vi "main.vi"() -> ()   [LabVIEW 2015]
uses:
  <vilib>/addons/InsightCM/MessageBus/MessageService/IcmMessageService.lvclass
  System/System.lvlib
  ConfigHelper/ConfigHelper.lvlib
  FileHandler/FileHandler.lvlib
  MainController/MainController.lvlib
  <vilib>/addons/Qbus/Qbus.lvclass
  CopyUtility/CopyUtility.lvlib
panel:
  in  "Control":bool
  out "System Status":string
  out "path":path
  out "error out":errorcluster
  out "Received Messages":i32(listbox)
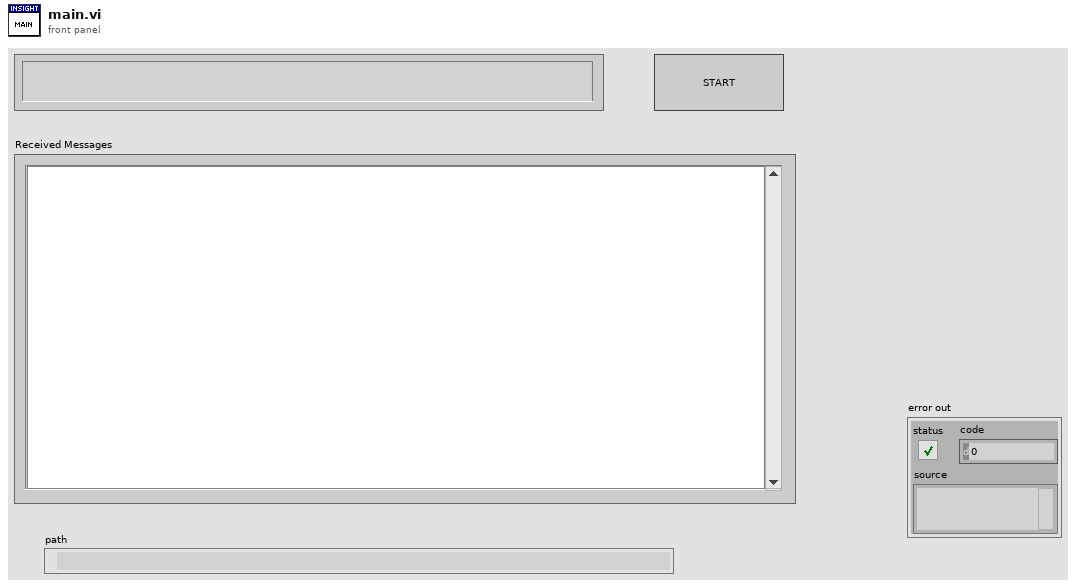
[diagram p1: front panel]
types:
  T1 = typedef "Message.ctl" = cluster{"Header":T2, "Body":u8[]}
  T2 = typedef "MessageHeader.ctl" = cluster{"MessageName":string, "Timestamp":i64, "CorrelationId":string, "ContentType":string, "RoutingKey":string, "Properties":T3[]}
  T3 = typedef "KeyValuePair.ctl" = cluster{"Key":string, "Value":string}
  T4 = typedef "StorageFileAvailableBroadcastBody.ctl" = cluster{"DeviceName":string, "Filepath":string}
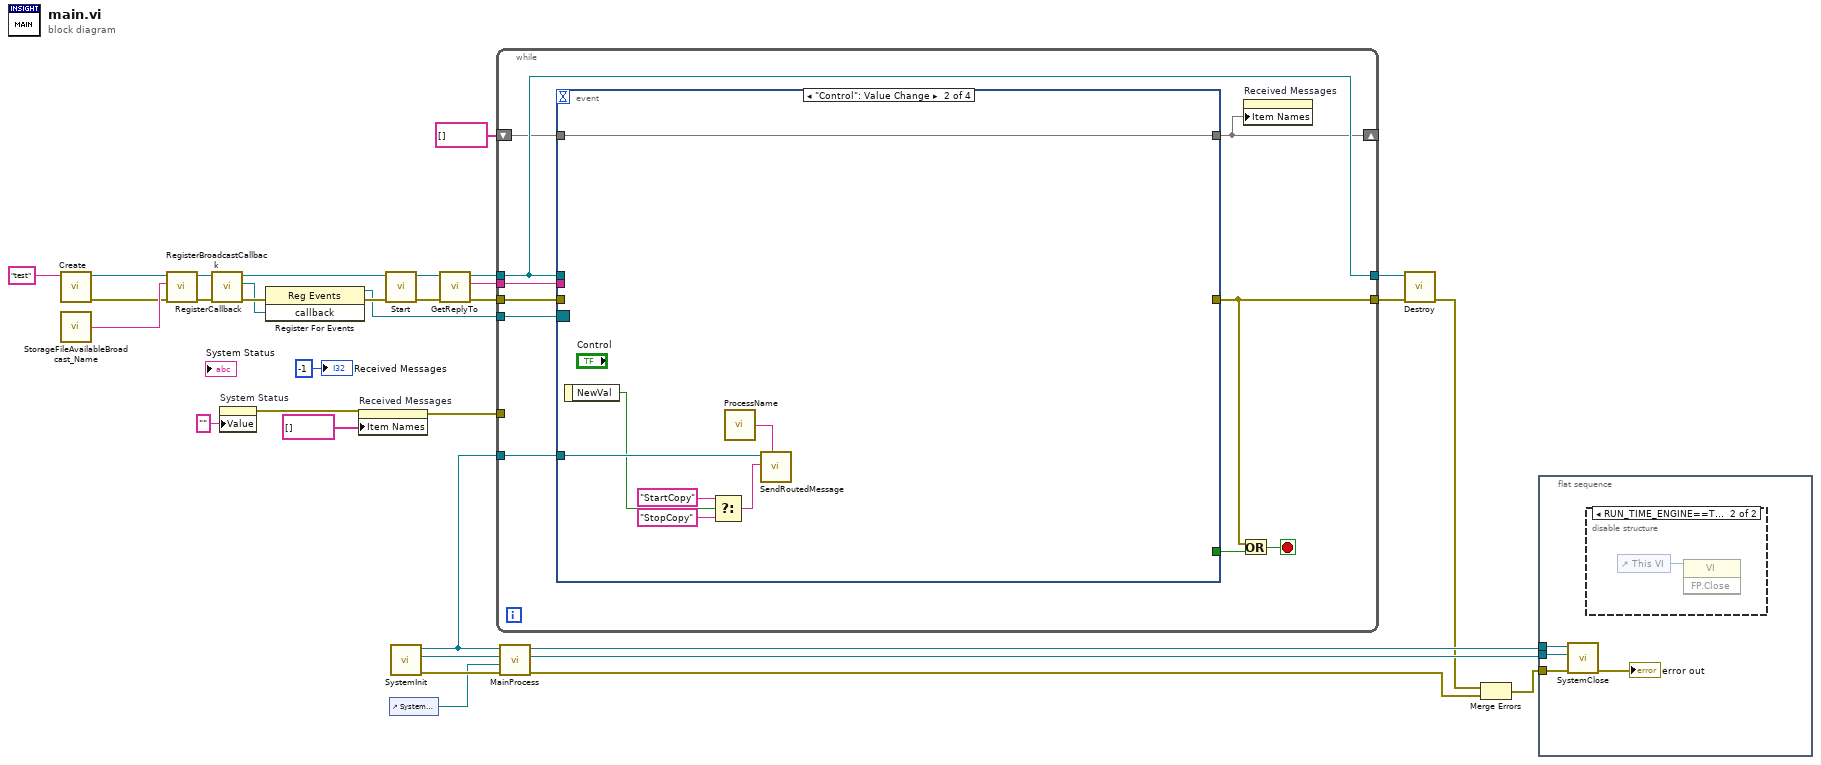
[diagram p0: block diagram]
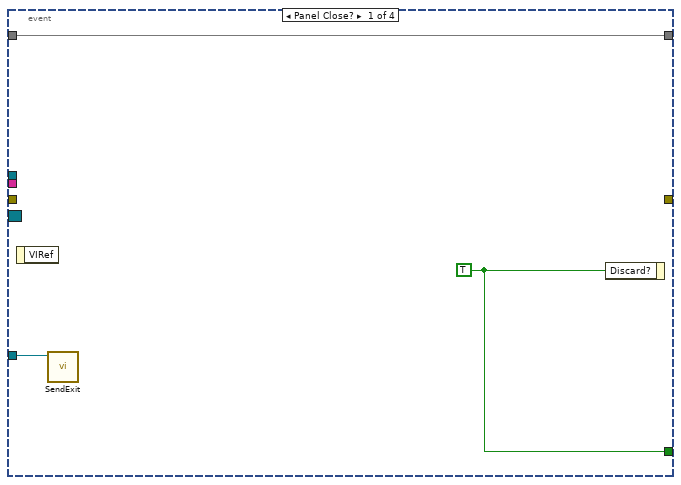
[diagram p3: hidden frame]
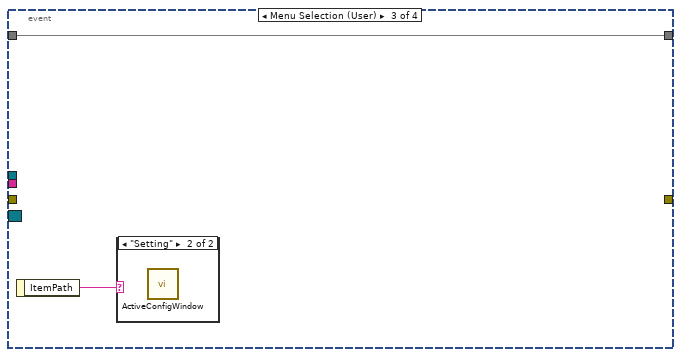
[diagram p4: hidden frame]
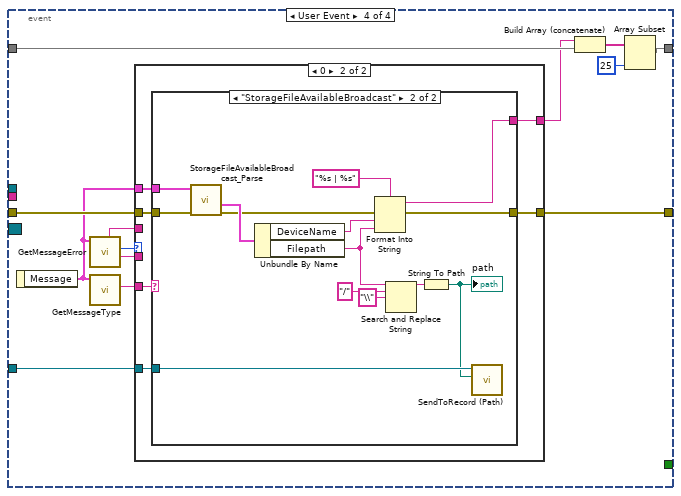
[diagram p6: hidden frame]
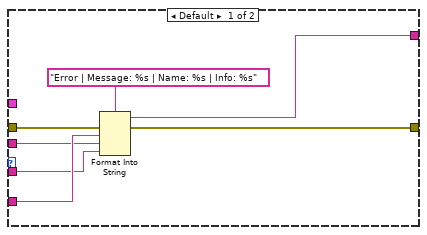
[diagram p7: hidden frame]
diagram:
  n1 = call <vilib>:"Create.vi"("service name"="test" ("Service Name")) -> ("error out"=w12:errorcluster, "service out"=w13:refnum<class "IcmMessageService.lvclass">)  [unwired: 9 in]
  n2 = call <vilib>:"StorageFileAvailableBroadcast_Name.vi"() -> ("MessageName"=w18:string)  [unwired: 5 in]
  n3 = call <vilib>:"RegisterBroadcastCallback.vi"("error in (no error)"=w12, "broadcast message"=w18, "service in"=w13) -> ("error out"=w17:errorcluster, "service out"=w16:refnum<class "IcmMessageService.lvclass">)  [unwired: 7 in]
  n4 = call <vilib>:"RegisterCallback.vi"("error in (no error)"=w17, "service in"=w16) -> ("error out"=w31:errorcluster, "callback"=w29:refnum<user-event>, "service out"=w32:refnum<class "IcmMessageService.lvclass">)  [unwired: 7 in]
  n5 = property on="System Status" class="Str"("Value"="" ("System Status")) -> (error out=w3:errorcluster)  [unwired: 2 in, 1 out]
  n6 = register-events(error in=w31, w29) -> (reference out=w28:refnum<event-registration>, error out=w30:errorcluster)  [unwired: 1 in]
  n7 = property on="Received Messages" class="LstBox (strict)"(error in=w3, "Item Names"=string[] []) -> (error out=w19:errorcluster)  [unwired: 1 in, 1 out]
  n8 = call <vilib>:"Start.vi"("error in (no error)"=w30, "service in"=w32) -> ("error out"=w24:errorcluster, "service out"=w26:refnum<class "IcmMessageService.lvclass">)  [unwired: 8 in]
  n9 = control-ref of="System Status"() -> (w1:refnum<vi>)
  n10 = call "SystemInit.vi"() -> ("error out"=w9:errorcluster, "Pound"=w11:refnum<class "Pound.lvclass">, "Qbus out"=w10:refnum<class "Qbus.lvclass">)  [unwired: 9 in]
  n11 = call <vilib>:"GetReplyTo.vi"("error in (no error)"=w24, "service in"=w26) -> ("error out"=w15:errorcluster, "reply to"=w23:string, "service out"=w25:refnum<class "IcmMessageService.lvclass">)  [unwired: 7 in]
  n12 = while {
    tunnel: w28 -> [w43]
    tunnel: w25 -> [w42]
    tunnel: [w42] -> w27
    tunnel: w23 -> [w41]
    shift-right: [w39] -> _
    shift-left: string[] [] -> [w40]
    tunnel: w19 -> [_]
    tunnel: w15 -> [w38]
    tunnel: [w36] -> w14
    tunnel: w10 -> [w34]
    stop <- w35 stop-if-true
    n13 = event shown="[1] \"Control\": Value Change" {
      selector: w43 -> [_ _ _ _]
      dyn-events: _ -> [_ _ _ _]
      timeout: _ -> [_ _ _ _]
      tunnel: [w46 _ _ _] -> w37
      tunnel: w42 -> [_ _ _ _]
      tunnel: w41 -> [_ _ _ _]
      tunnel: [w45 w53 w55 w67] -> w39
      tunnel: w40 -> [w45 w53 w55 w66]
      tunnel: w38 -> [_ _ _ w59]
      tunnel: [_ _ _ w58] -> w36
      tunnel: w34 -> [w44 w52 _ w56]
      event Panel Close? {
        w46 = TRUE ("Discard?")
        n14 = event-data() -> ()  [unwired: 1 in, 1 out]
        n15 = call "SendExit.vi"("Qbus in"=w44) -> ()  [unwired: 9 in, 2 out]
        n16 = event-data("Discard?"=w46) -> ()  [unwired: 1 in, 1 out]
      }
      event "Control": Value Change {
        n17 = event-data() -> ("NewVal"=w51:bool)  [unwired: 1 in]
        n18 = Select(t="StartCopy", s=w51, f="StopCopy") -> (s? t:f=w48:string)
        n19 = call "ProcessName.vi"() -> ("process name"=w47:string)  [unwired: 5 in]
        n20 = call <vilib>:"SendRoutedMessage.vi"("listener process"=w47, "message name"=w48, "Qbus in"=w52) -> ()  [unwired: 7 in, 2 out]
      }
      event Menu Selection (User) {
        n21 = event-data() -> ("ItemPath"=w54:string)  [unwired: 1 in]
        n22 = case shown="\"Setting\"" w54 {
          frame Default {
          }
          frame "Setting" {
            n23 = call "ActiveConfigWindow.vi"() -> ()  [unwired: 12 in]
          }
        }
      }
      event User Event {
        n24 = event-data() -> ("Message"=w57:T1)  [unwired: 1 in]
        n25 = call <vilib>:"GetMessageError.vi"("message in"=w57) -> ("error info"=w60:string, "error code"=w62:i32, "error name"=w61:string)  [unwired: 7 in, 1 out]
        n26 = call <vilib>:"GetMessageType.vi"("message in"=w57) -> ("message name"=w64:string)  [unwired: 9 in, 1 out]
        n27 = case shown="0" w62 {
          tunnel: w64 -> [w74 w81]
          tunnel: [w71 w80] -> w63
          tunnel: w61 -> [w73 _]
          tunnel: w60 -> [w72 _]
          tunnel: w59 -> [w70 w79]
          tunnel: [w69 w78] -> w58
          tunnel: w57 -> [_ w77]
          tunnel: w56 -> [_ w76]
          frame Default {
            n28 = Format Into String(format string="Error | Message: %s | Name: %s | Info: %s", error in=w70, w74, w73, w72) -> (resulting string=w71:string, error out=w69:errorcluster)  [unwired: 1 in]
          }
          frame 0 {
            n29 = case shown="\"StorageFileAvailableBroadcast\"" w81 {
              selector: w81 -> [w83 _]
              tunnel: [w83 w95] -> w80
              tunnel: w79 -> [w82 w92]
              tunnel: [w82 w93] -> w78
              tunnel: w77 -> [_ w90]
              tunnel: w76 -> [_ w85]
              frame Default {
              }
              frame "StorageFileAvailableBroadcast" {
                n30 = call <vilib>:"StorageFileAvailableBroadcast_Parse.vi"("error in (no error)"=w92, "Message"=w90) -> ("error out"=w91:errorcluster, "Body"=w94:T4)  [unwired: 6 in, 2 out]
                n31 = Unbundle By Name(w94) -> ("DeviceName"=w96:string, "Filepath"=w89:string)
                n32 = Format Into String(format string="%s | %s", error in=w91, w96, w89) -> (resulting string=w95:string, error out=w93:errorcluster)  [unwired: 1 in]
                n33 = Search and Replace String(input string=w89, search string="/", replace string="\\" ("replace string (\"\")")) -> (result string=w88:string)  [unwired: 5 in, 3 out]
                n34 = String To Path(string=w88) -> (path=w84:path)
                "path" <- w84
                n35 = call "SendToRecord (Path).vi"("Path"=w84, "Qbus in"=w85) -> ()  [unwired: 9 in, 1 out]
              }
            }
          }
        }
        n36 = Build Array (concatenate)(w63, w66) -> (w68:string[])
        n37 = Array Subset(array=w68, length=25) -> (w67:string[])  [unwired: 1 in]
      }
    }
    n38 = Or(x=w36, y=w37) -> (x .or. y?=w35:bool)
    n39 = property on="Received Messages" class="LstBox (strict)"("Item Names"=w39) -> ()  [unwired: 2 in, 2 out]
  }
  n40 = call "MainProcess.vi"("error in (no error)"=w9, "System Status Ref."=w1, "pound in"=w11, "qbus in"=w10) -> ("error out"=w5:errorcluster, "Pound"=w7:refnum<class "Pound.lvclass">, "Qbus out"=w8:refnum<class "Qbus.lvclass">)  [unwired: 5 in]
  n41 = call <vilib>:"Destroy.vi"("error in (no error)"=w14, "service in"=w27) -> ("error out"=w6:errorcluster)  [unwired: 9 in]
  n42 = Merge Errors(w6, w5) -> (w4:errorcluster)
  n43 = flat-sequence {
    tunnel: w8 -> [w101]
    tunnel: w7 -> [w100]
    tunnel: w4 -> [w99]
    frame #0 {
      n44 = call "SystemClose.vi"("error in (no error)"=w99, "Pound"=w100, "Qbus"=w101) -> ("error out"=→"error out":errorcluster)  [unwired: 8 in]
      n45 = disable-structure shown="RUN_TIME_ENGINE==True" {
        frame condition #0 (active) {
        }
        frame condition #1 {
          n46 = control-ref of="This VI"() -> (w102:refnum<vi>)
          n47 = invoke class="VI" method="FP.Close"(reference=w102) -> ()  [unwired: 2 in, 3 out]
        }
      }
    }
  }
  "Received Messages" <- -1 ("Received Messages")
